vi "Lab 2.vi"() -> ()   [LabVIEW 2021]
uses:
  <vilib>/express/express arith-compare/Formula/XNode/ExpressFormulaBlockNode.xnode
panel:
  in  "Tab Control":enum32{"Page 1", "Page 2"}(tab)
  out "Area - Method 3":dbl
  out "Area - Method 2":dbl
  out "Volume - Method 3":dbl
  out "Volume - Method 2":dbl
  in  "stop":bool
  out "Area - Method 1":dbl
  out "Volume - Method 1":dbl
  in  "Radius":dbl
  out "String":string
  out "Answer - Method  3":dbl
  out "Answer - Method 2":dbl
  out "Answer - Method 1":dbl
  in  "y":dbl
  in  "x":dbl
  # "2xy^2+4xy+8"
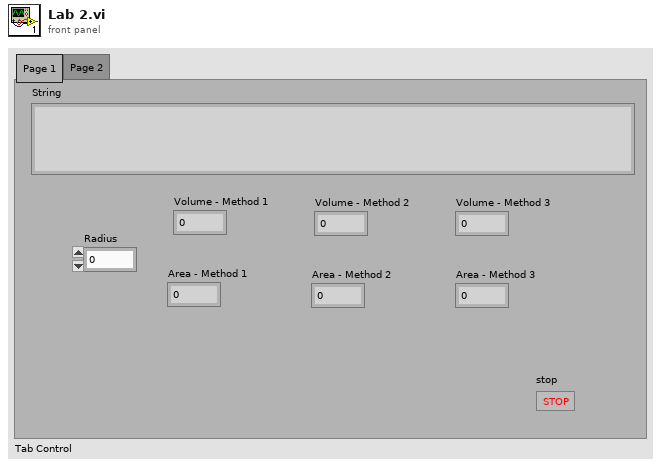
[diagram p1: front panel]
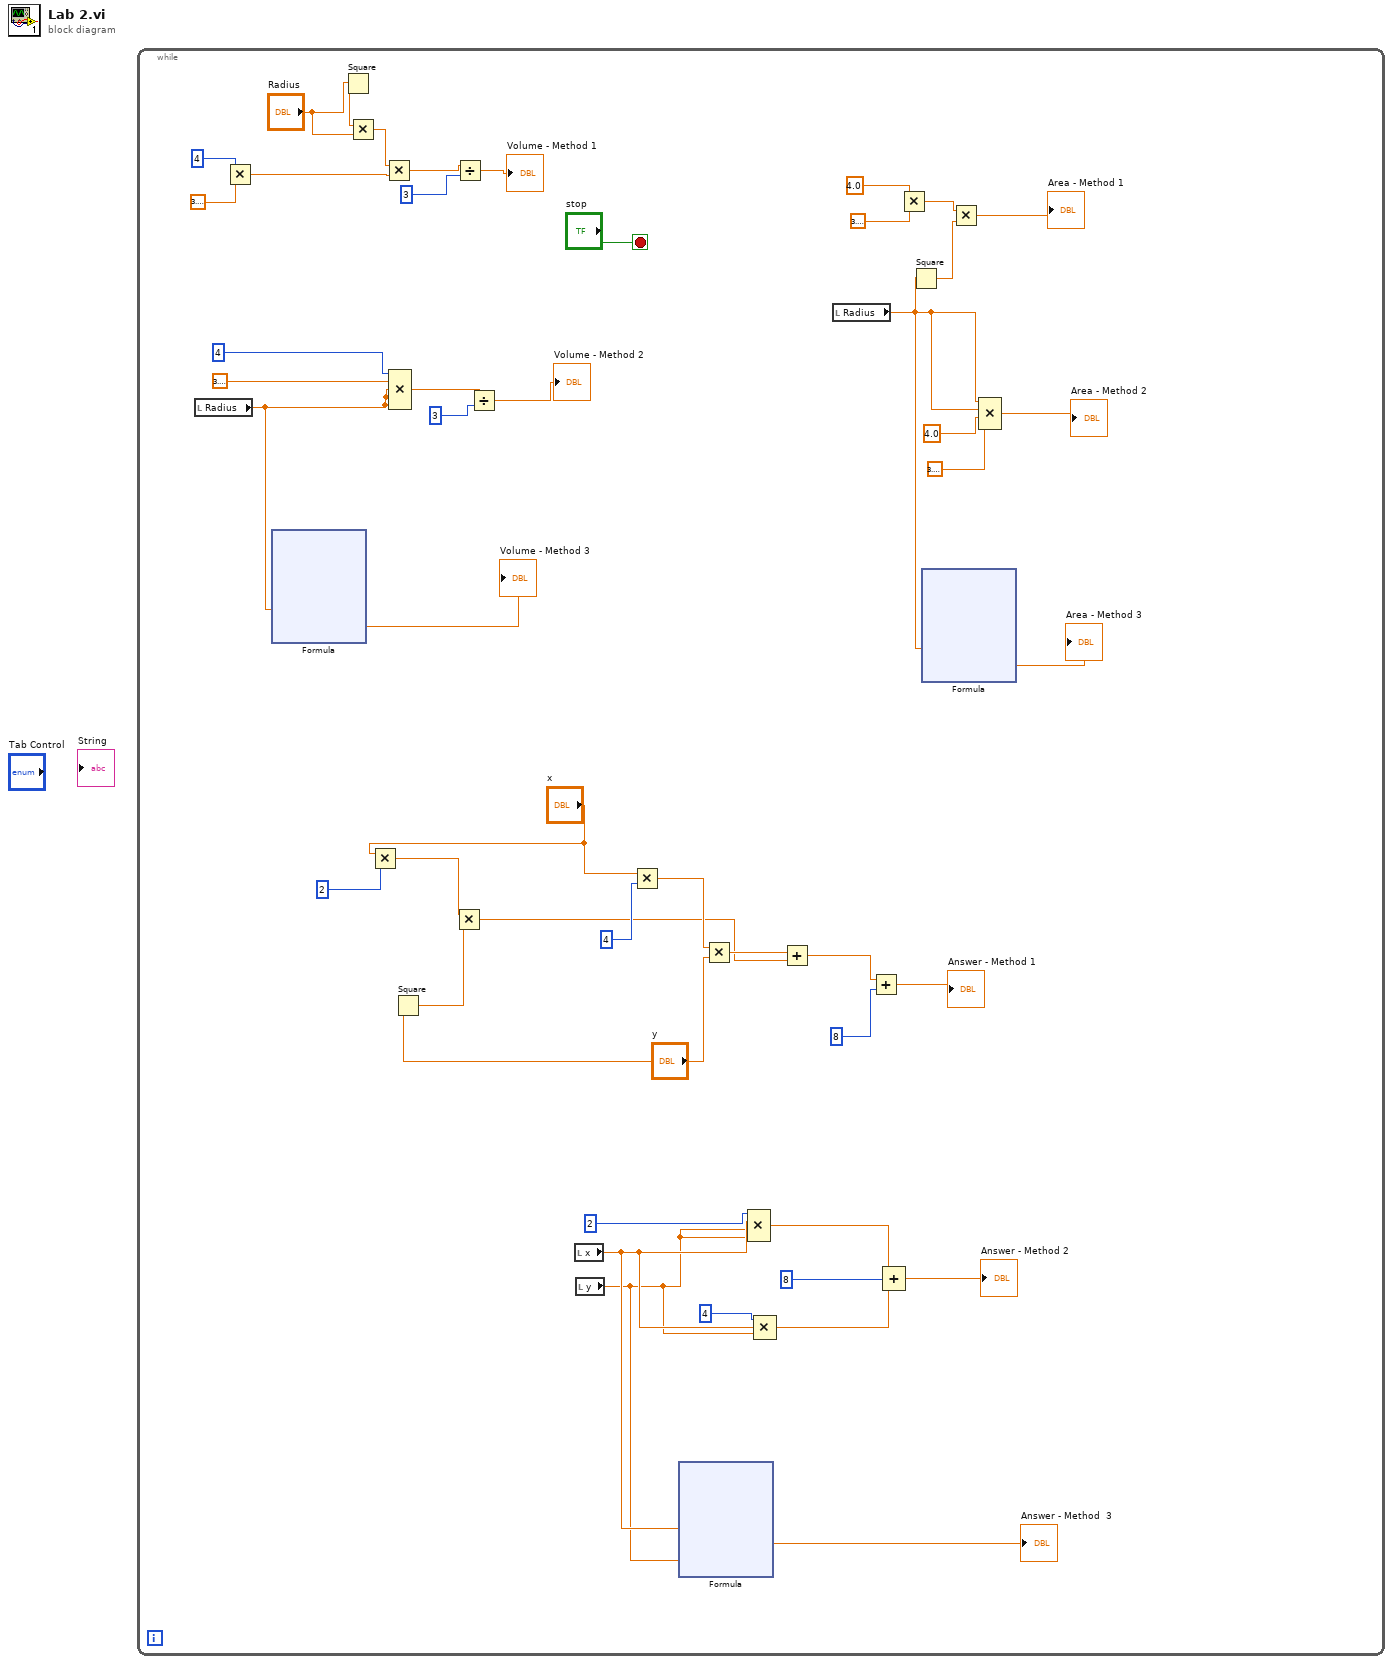
[diagram p0: block diagram]
diagram:
  n1 = while {
    stop <- "stop" stop-if-true
    n2 = local read "Radius"() -> (w32:dbl)
    n3 = Multiply(x=4, y=3.141592653589793) -> (x*y=w43:dbl)
    n4 = xnode "Formula"("r"=w32) -> ("Result"=→"Volume - Method 3":dbl)  [unwired: 1 in, 1 out]
    n5 = Square(x="Radius") -> (x^2=w46:dbl)
    n6 = Multiply(x=w46, y="Radius") -> (x*y=w44:dbl)
    n7 = Multiply(x="x", y=2) -> (x*y=w20:dbl)
    n8 = Multiply(x=w44, y=w43) -> (x*y=w41:dbl)
    n9 = Compound Arithmetic op=MULTIPLY(4, 3.141592653589793, w32, w32, w32) -> (w37:dbl)
    n10 = Square(x="y") -> (x^2=w19:dbl)
    n11 = Multiply(x=w20, y=w19) -> (x*y=w13:dbl)
    n12 = Divide(x=w41, y=3) -> (x/y=→"Volume - Method 1":dbl)
    n13 = Divide(x=w37, y=3) -> (x/y=→"Volume - Method 2":dbl)
    n14 = local read "x"() -> (w3:dbl)
    n15 = local read "y"() -> (w2:dbl)
    n16 = Multiply(x="x", y=4) -> (x*y=w16:dbl)
    n17 = xnode "Formula"("x"=w3, "y"=w2) -> ("Result"=→"Answer - Method  3":dbl)  [unwired: 1 in, 1 out]
    n18 = Multiply(x=w16, y="y") -> (x*y=w14:dbl)
    n19 = Compound Arithmetic op=MULTIPLY(2, w3, w2, w2) -> (w5:dbl)
    n20 = Compound Arithmetic op=MULTIPLY(4, w3, w2) -> (w6:dbl)
    n21 = Add(x=w14, y=w13) -> (x+y=w12:dbl)
    n22 = local read "Radius"() -> (w23:dbl)
    n23 = Add(x=w12, y=8) -> (x+y=→"Answer - Method 1":dbl)
    n24 = Compound Arithmetic op=ADD(w5, 8, w6) -> (→"Answer - Method 2":dbl)
    n25 = Multiply(x=4.0, y=3.141592653589793) -> (x*y=w28:dbl)
    n26 = Square(x=w23) -> (x^2=w31:dbl)
    n27 = xnode "Formula"("r"=w23) -> ("Result"=→"Area - Method 3":dbl)  [unwired: 1 in, 1 out]
    n28 = Multiply(x=w28, y=w31) -> (x*y=→"Area - Method 1":dbl)
    n29 = Compound Arithmetic op=MULTIPLY(w23, w23, 4.0, 3.141592653589793) -> (→"Area - Method 2":dbl)
  }
